vi "DPDD2dll.vi"(8 "error in (no error)":errorcluster, 9 "z":dbl[](array[numeric]), 10 "D":dbl, 11 "t":dbl) -> (0 "error out":errorcluster, 3 "d2PdD2 out":dbl)   [LabVIEW 2016]
doc: "subroutine DPDD2dll(t, D, z, d2pdd2)\n\nCompute second partial derivative of pressure w.r.t. density at constant temperature as a function of temperature,\ndensity, and composition. See warning in suroutines THERM or ALLPROPS.\n\nINPUTS:\nt -- Temperature [K]\nD -- Molar density [mol/L]\nz -- Composition (array of mole fractions)\n\nOUTPUTS:\nd2pdd2 -- d^2P/dD^2 [kPa-L^2/mol^2]"
uses:
  REFPROP.DLL
panel:
  # "REFPROP-DPDD2dll.vi"
  # "void  DPDD2dll(double *t, double *D, double *z, double *d2pdd2)"
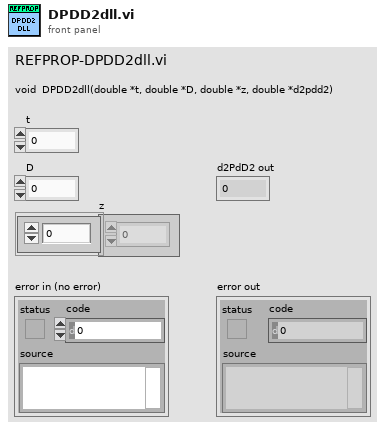
[diagram p1: front panel]
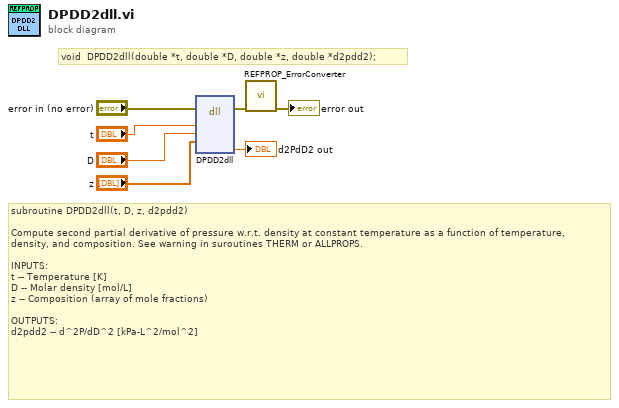
[diagram p0: block diagram]
diagram:
  # "void  DPDD2dll(double *t, double *D, double *z, double *d2pdd2);"
  # "subroutine DPDD2dll(t, D, z, d2pdd2)\n\nCompute second partial derivative of pressure w.r.t. density at constant temperature as a function of temperature,\ndensity, and composition. See warning in suroutines THERM or ALLPROPS.\n\nINPUTS:\nt -- Temperature [K]\nD -- Molar density [mol/L]\nz -- Composition (array of mole fractions)\n\nOUTPUTS:\nd2pdd2 -- d^2P/dD^2 [kPa-L^2/mol^2]"
  n1 = dll-call lib="S:/009 - Testing/02 - Performance Testing/REFPROP/REFPROP.*" fn="DPDD2dll"(error in="error in (no error)", "t"="t", "D"="D", "z"="z") -> (error out=w3:errorcluster, "d2pdd2"=→"d2PdD2 out":dbl)  [unwired: 7 in, 1 out]
  n2 = call "REFPROP_ErrorConverter.vi"("error in (no error)"=w3) -> ("error out"=→"error out":errorcluster)  [unwired: 10 in]
